vi "NiFpga_HdlFifo32_ReadI8.vi"(6 "timeout":u32, 7 "error in (no error)":errorcluster, 8 "number of elements":i32, 9 "fifo number":u32, 10 "fpga vi reference in":refnum<k20>) -> (0 "error out":errorcluster, 1 "elements remaining":u64, 2 "data out":i8[](array[numeric]), 3 "fpga vi reference out":refnum<k20>)   [LabVIEW 2023]
doc: "Dynamically reads the register at the provided offset. Set check for errors to true to check for errors such as if the register offset is invalid or if the register is running in an external clock domain that might not be running."
uses:
  NiFpga.dll
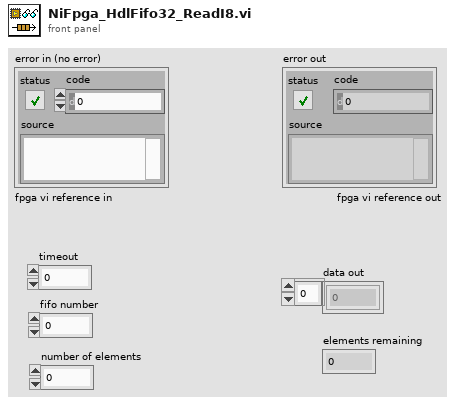
[diagram p1: front panel]
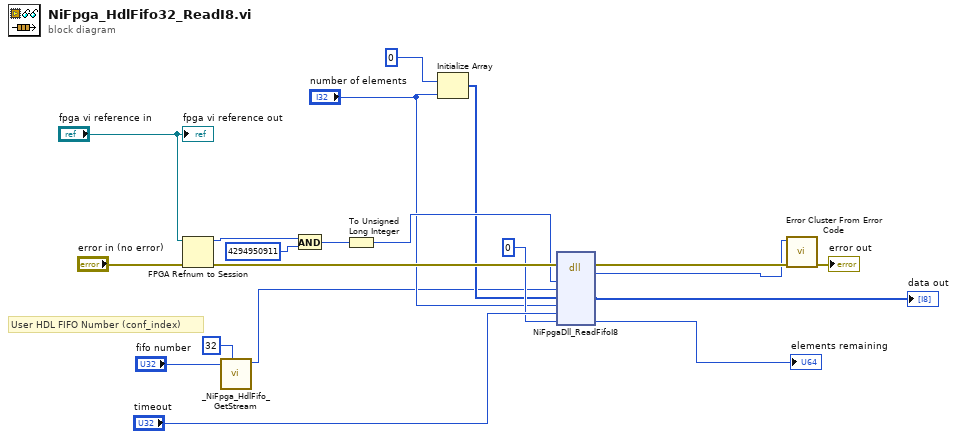
[diagram p0: block diagram]
diagram:
  # "User HDL FIFO Number (conf_index)"
  n1 = FPGA Refnum to Session(4:"error in (no error)", 7:"fpga vi reference in") -> (0:w15:errorcluster, 3:w17:u64)
  n2 = call "_NiFpga_HdlFifo_GetStream.vi"("NUM_DMA_CHANNELS"=u32 32, "Fifo Number"="fifo number") -> ("Fifo Stream"=w2:u32)  [unwired: 9 in]
  n3 = And(x=w17, y=u64 4294950911) -> (x .and. y?=w10:u64)
  n4 = To Unsigned Long Integer(number=w10) -> (unsigned 32bit integer=w9:u32)
  n5 = Initialize Array(i8 0, "number of elements") -> (w5:i8[])
  n6 = dll-call lib="NiFpga.*" fn="NiFpgaDll_ReadFifoI8"(error in=w15, "session"=w9, "fifo"=w2, "data"=w5, "numberOfElements"="number of elements", "timeout"="timeout", "elementsRemainining"=u64 0 ("emptyElementsRemainining")) -> (error out=w14:errorcluster, "return type"=w13:i32, "data"=→"data out":i8[], "elementsRemainining"=→"elements remaining":u64)  [unwired: 6 in, 1 out]
  n7 = call <vilib>:"Error Cluster From Error Code.vi"("error in (no error)"=w14, "error code (0)"=w13) -> ("error out"=→"error out":errorcluster)  [unwired: 7 in]
  "fpga vi reference out" <- "fpga vi reference in"
